vi "TaskProps.vi"(5 "task in":refnum<k24>, 7 "error in (no error)":errorcluster) -> (0 "task out":refnum<k24>, 1 "NumberOfChannels":u32, 2 "Done":bool, 3 "error out":errorcluster, 4 "DeviceName":string)   [LabVIEW 2010]
uses:
  C:/Program Files/National Instruments/LabVIEW 2010/vi.lib/ULx/ULx_LV.dll
  Program Files/National Instruments/LabVIEW 2010/vi.lib/ULx/ULx_LV.dll
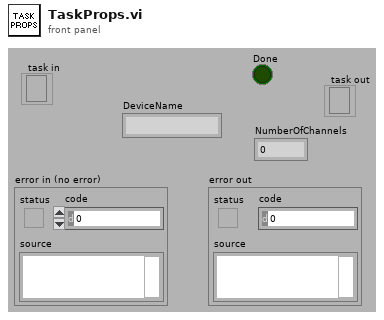
[diagram p1: front panel]
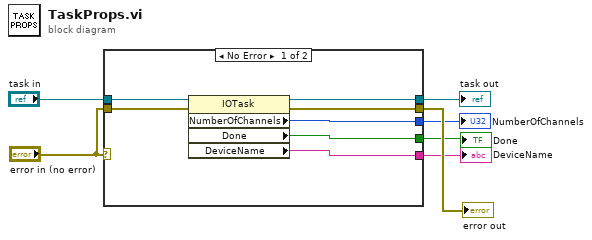
[diagram p0: block diagram]
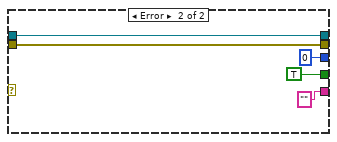
[diagram p2: hidden frame]
diagram:
  n1 = case shown="No Error" "error in (no error)" {
    tunnel: "task in" -> [w14 w19]
    tunnel: "error in (no error)" -> [w11 w18]
    tunnel: [w13 w19] -> w6
    tunnel: [w12 w18] -> w5
    tunnel: [w10 u32 0 ("NumberOfChannels")] -> w3
    tunnel: [w9 TRUE ("Done")] -> w2
    tunnel: [w8 "" ("DeviceName")] -> w1
    frame No Error {
      n2 = property class="IOTask"(reference=w14, error in=w11) -> (reference out=w13:refnum<k24>, error out=w12:errorcluster, "NumberOfChannels"=w10:u32, "Done"=w9:bool, "DeviceName"=w8:string)
    }
    frame Error {
    }
  }
  "task out" <- w6
  "error out" <- w5
  "NumberOfChannels" <- w3
  "Done" <- w2
  "DeviceName" <- w1
